vi "ExtndKalman_CardiacModel.vi"(0 "Sample Interval (sec)":dbl, 1 "State_n_n":T2, 2 "State_n_n Var":T3, 5 "y_n (hemodynamic value)":dbl, 7 "Noise Var (r)":dbl, 9 "P_n_1":T1, 11 "w_bar_ca":dbl, 12 "w_bar_r":dbl, 13 "Alpha_c":dbl, 14 "Alpha_r":dbl) -> (4 "Output State":T2, 10 "Trend":dbl, 15 "P_n_n_1":T1)   [LabVIEW 2019]
uses:
  <vilib>/Analysis/Matrix/Datatypes/RealMatrix.ctl
  <vilib>/Analysis/baseanly.llb/Real A x B.vi
  <vilib>/Analysis/baseanly.llb/A x Vector.vi
  <vilib>/Analysis/Matrix/Numeric/Add/Add (Elementwise) - RM,R.vi
  <vilib>/Analysis/baseanly.llb/Real Inverse Matrix.vi
  <vilib>/Analysis/Matrix/Numeric/Subtract/Subtract - RM,RM.vi
  <vilib>/Analysis/Matrix/Numeric/Add/Add - RM,RM.vi
  <vilib>/Analysis/Matrix/NI_Matrix.lvlib
  <vilib>/Analysis/NI_AALBase.lvlib
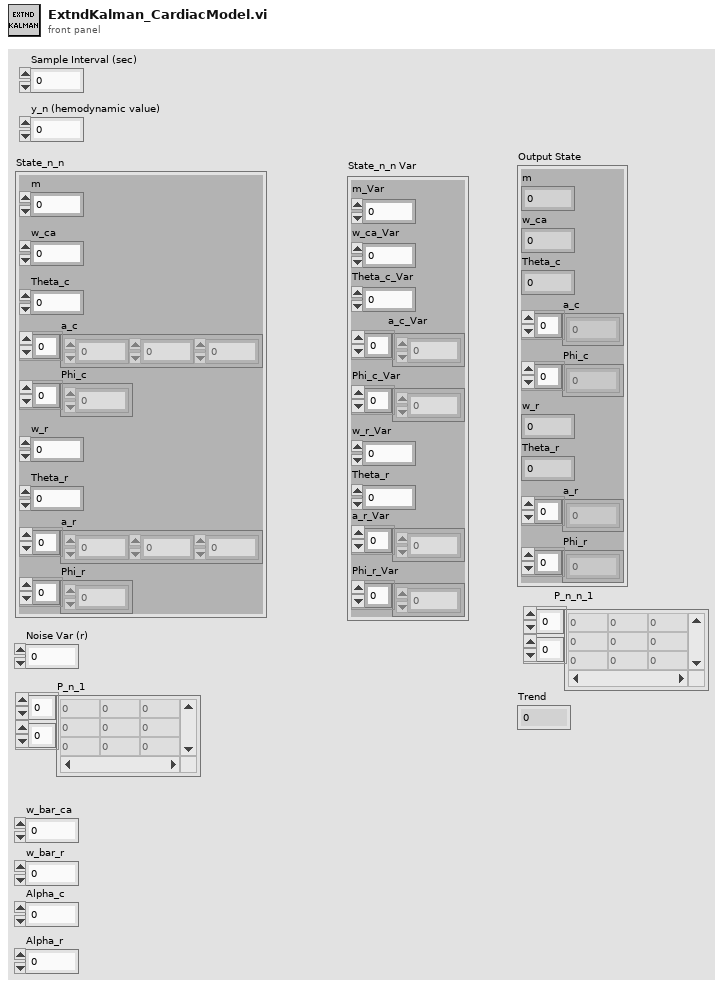
[diagram p1: front panel]
types:
  T1 = typedef "NI_Matrix.lvlib/RealMatrix.ctl" = dbl[][]
  T2 = cluster{"m":dbl, "w_ca":dbl, "Theta_c":dbl, "a_c":dbl[], "Phi_c":dbl[], "w_r":dbl, "Theta_r":dbl, "a_r":dbl[], "Phi_r":dbl[]}
  T3 = cluster{"m_Var":dbl, "w_ca_Var":dbl, "Theta_c_Var":dbl, "a_c_Var":dbl[], "Phi_c_Var":dbl[], "w_r_Var":dbl, "Theta_r":dbl, "a_r_Var":dbl[], "Phi_r_Var":dbl[]}
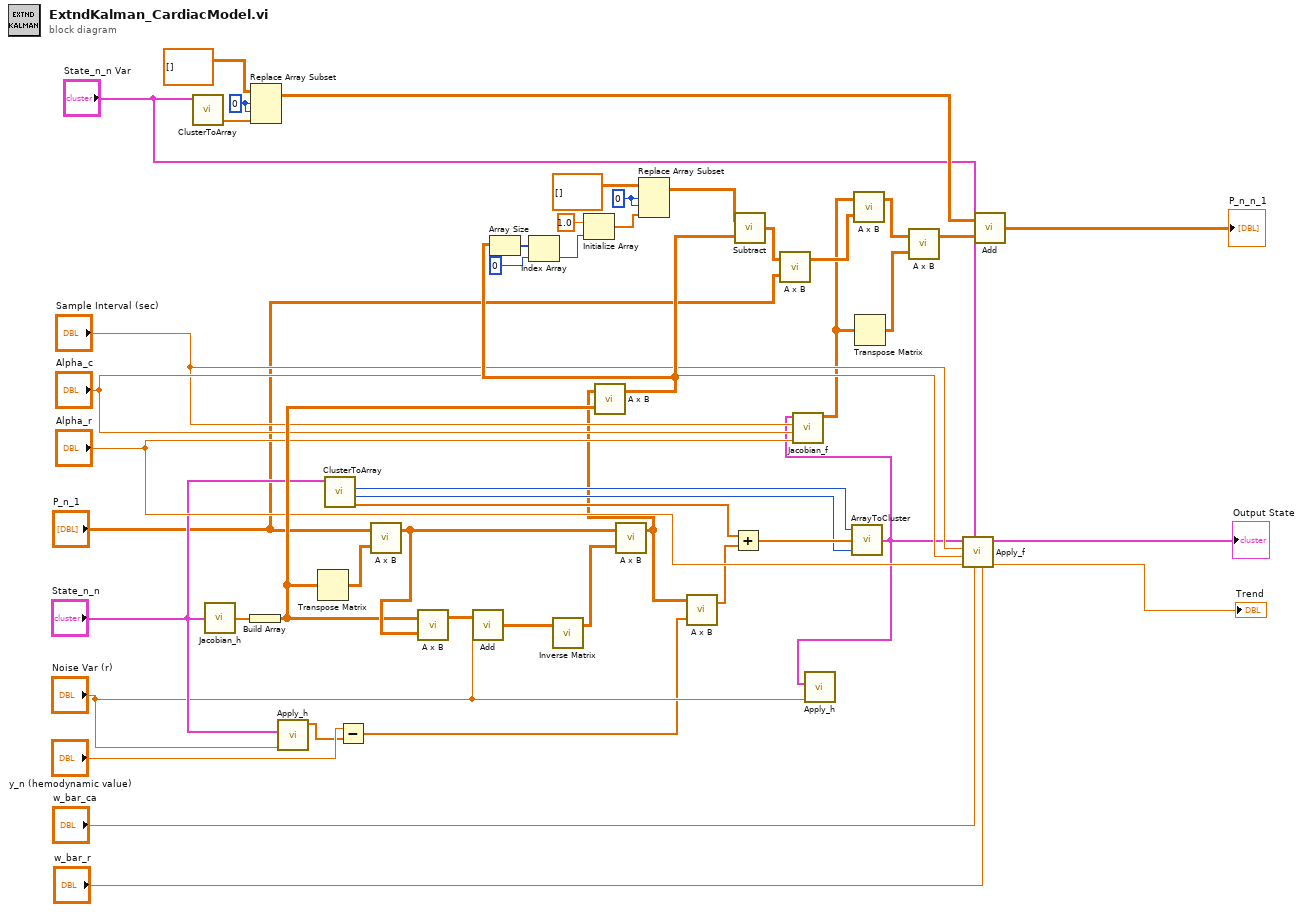
[diagram p0: block diagram]
diagram:
  w22 = 0 ("disabled index (row)")
  w36 = 0 ("disabled index (row)")
  n1 = call "ClusterToArray.vi"("State_n_n"="State_n_n Var") -> ("State Array"=w21:dbl[])  [unwired: 2 out]
  n2 = call "Jacobian_h.vi"("State"="State_n_n") -> ("J_h(H_n)"=w48:dbl[])
  n3 = Build Array(w48) -> (w32:T1)
  n4 = Replace Array Subset(array=T1 [] ("matrix"), new element=w21, index (row)=w22, index (col)=w22) -> (w20:T1)
  n5 = call "Apply_h.vi"("Noise Var"="Noise Var (r)", "Input State"="State_n_n") -> ("h(x)"=w41:dbl[])  [unwired: 2 in, 3 out]
  n6 = Transpose Matrix(1:w32) -> (0:w47:T1)
  n7 = call "ClusterToArray.vi"("State_n_n"="State_n_n") -> ("State Array"=w40:dbl[], "N_r"=w37:i32, "N_c"=w38:i32)
  n8 = Subtract(x="y_n (hemodynamic value)", y=w41) -> (x-y=w6:dbl[])
  n9 = call-poly <vilib>:"A x B.vi"("B"=w47, "A"="P_n_1") -> ("A x B"=w45:T1)  [unwired: 1 out]
  n10 = call-poly <vilib>:"A x B.vi"("B"=w45, "A"=w32) -> ("A x B"=w43:T1)  [unwired: 1 out]
  n11 = call-poly <vilib>:"Add.vi"("Real Scalar c"="Noise Var (r)", "Real Matrix A"=w43) -> ("A + c"=w46:T1)
  n12 = call-poly <vilib>:"Inverse Matrix.vi"("Input Matrix"=w46) -> ("Inverse Matrix"=w44:T1)  [unwired: 1 in, 1 out]
  n13 = call-poly <vilib>:"A x B.vi"("B"=w44, "A"=w45) -> ("A x B"=w7:T1)  [unwired: 1 out]
  n14 = call-poly <vilib>:"A x B.vi"("B"=w32, "A"=w7) -> ("A x B"=w28:T1)  [unwired: 1 out]
  n15 = Array Size(array=w28) -> (size(s)=w8:i32[])
  n16 = Index Array(array=w8, index=0) -> (element=w30:i32)
  n17 = Initialize Array(1.0 ("element"), w30) -> (w34:dbl[])
  n18 = Replace Array Subset(array=T1 [] ("matrix"), new element=w34, index (row)=w36, index (col)=w36) -> (w29:T1)
  n19 = call-poly <vilib>:"A x B.vi"("Vector"=w6, "A"=w7) -> ("A x Vector"=w5:dbl[])  [unwired: 1 out]
  n20 = Add ("Add.vi")(x=w40, y=w5) -> (x+y=w39:dbl[])
  n21 = call-poly <vilib>:"Subtract.vi"("Real Matrix B"=w28, "Real Matrix A"=w29) -> ("A - B"=w27:T1)
  n22 = call-poly <vilib>:"A x B.vi"("B"="P_n_1", "A"=w27) -> ("A x B"=w26:T1)  [unwired: 1 out]
  n23 = call "ArrayToCluster.vi"("N_r"=w37, "State Array"=w39, "N_c"=w38) -> ("State Cluster"=w9:T2)
  n24 = call "Jacobian_f.vi"("Alpha_r"="Alpha_r", "Alpha_c"="Alpha_c", "Sample Interval (sec)"="Sample Interval (sec)", "Input State"=w9) -> ("J_f"=w2:T1)  [unwired: 7 in]
  n25 = call "Apply_h.vi"("Noise Var"="Noise Var (r)", "Input State"=w9) -> ()  [unwired: 2 in, 4 out]
  n26 = call-poly <vilib>:"A x B.vi"("B"=w26, "A"=w2) -> ("A x B"=w25:T1)  [unwired: 1 out]
  n27 = Transpose Matrix(1:w2) -> (0:w24:T1)
  n28 = call-poly <vilib>:"A x B.vi"("B"=w24, "A"=w25) -> ("A x B"=w19:T1)  [unwired: 1 out]
  n29 = call "Apply_f.vi"("w_bar_r"="w_bar_r", "w_bar_ca"="w_bar_ca", "Input State Var"="State_n_n Var", "Alpha_r"="Alpha_r", "Alpha_c"="Alpha_c", "T"="Sample Interval (sec)", "Input State"=w9) -> ("Trend"=→"Trend":dbl, "Output State"=→"Output State":T2)  [unwired: 3 in]
  n30 = call-poly <vilib>:"Add.vi"("Real Matrix B"=w19, "Real Matrix A"=w20) -> ("A + B"=→"P_n_n_1":T1)
